vi "Global Variable.vi"() -> ()   [LabVIEW 2025]
panel:
  out "Winner":i32
  out "Show_hover":bool
  in  "Player":i32
  in  "Board":i32[][](array[numeric])
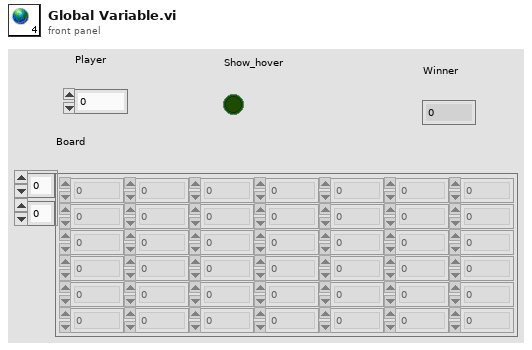
[diagram p1: front panel]
diagram:
